vi "RolloverCounter.vi"(7 "RolloverNum":u32, 9 "Increment":bool=TRUE, 10 "In":u32) -> (1 "Rollover":bool, 2 "Count":u32, 5 "Last":bool)   [LabVIEW 2011]
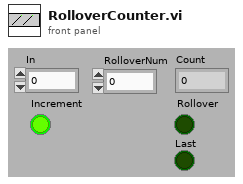
[diagram p1: front panel]
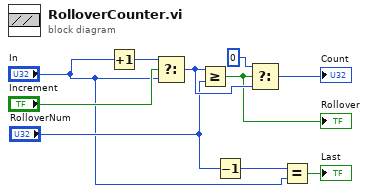
[diagram p0: block diagram]
diagram:
  n1 = Increment(x="In") -> (x+1=w9:u32)
  n2 = Select(t=w9, s="Increment", f="In") -> (s? t:f=w8:u32)
  n3 = Greater Or Equal?(x=w8, y="RolloverNum") -> (x >= y?=w6:bool)
  "Rollover" <- w6
  n4 = Decrement(x="RolloverNum") -> (x-1=w3:u32)
  n5 = Select(t=i16 0, s=w6, f=w8) -> (s? t:f=→"Count":u32)
  n6 = Equal?(x=w3, y="In") -> (x = y?=→"Last":bool)
